vi "Main_MHM01.vi"() -> ()   [LabVIEW 2013]
uses:
  <vilib>/Platform/TimedLoop/XDataNode/timing_clust.ctl
  <vilib>/Platform/TimedLoop/XDataNode/nitl_modes.ctl
  <vilib>/Platform/TimedLoop/XDataNode/wakeup.ctl
  <vilib>/platform/TimedLoop/XDataNode/XDataNode.xnode
  <vilib>/Platform/TimedLoop/XDataNode/XDNodeRunTimeDep.lvlib
panel:
  out "Export Folder Path":path
  in  "DO select":dbl[](array[numeric])
  in  "Names legend":string[](array[string])=["s1", "s2"]
  out "Unit display A":dbl[][](graph)=[[528.1875, 527.4375, 528.1875, 527.25, 525.75, 520.125, 579.0, 800.8125, 526.6875, 524.25, 525.0, 525.1875]]
  in  "Period (ms)":i64=1000
  out "DO indicator":bool[](array[boolean])
  in  "AI select":dbl[](array[numeric])
  out "Sample number":u32
  in  "Stop Button":bool
  # "SELECT DO AND AI FOR EACH SENSOR"
  # "DATA folder in VI location must be created manually"
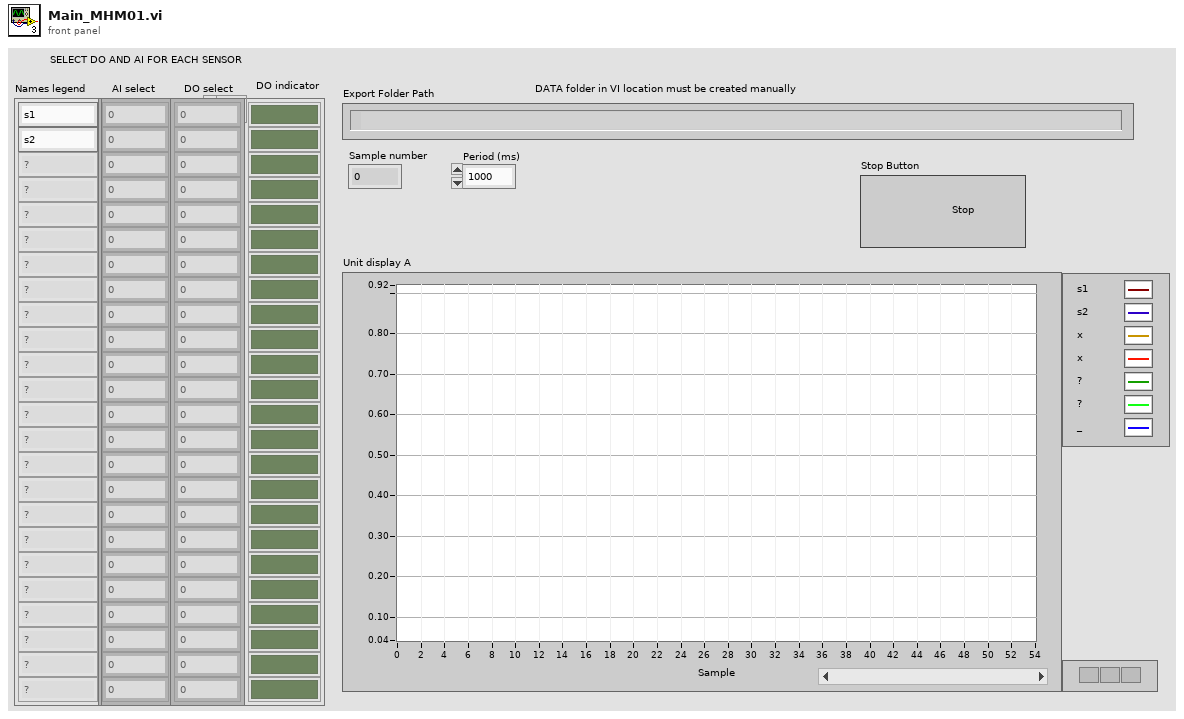
[diagram p1: front panel]
types:
  T1 = typedef "XDNodeRunTimeDep.lvlib/timing_clust.ctl" = cluster{"Expected End [f-1]":u64, "Actual End [f-1]":u64, "Finished Late? [f-1]":bool, "Expected End [i-1]":u64, "Actual End [i-1]":u64, "Finished Late? [i-1]":bool, "Expected Start [i]":u64, "Actual Start [i]":u64, "Expected Start [f]":u64, "Actual Start [f]":u64, "Source Name":string, "Structure Name":string, "Period":i64, "Deadline":i64, "Offset":i64, "Start":i64, "Priority":i32, "Timeout":i32, "Mode":T2, "Wakeup Reason":T3, "Error":errorcluster, "Source Type":string, "Secondary Source Type":string, "Global End Time":u64, "Global Start Time":u64, "Frame Duration":u64, "Iteration Duration":u64, "Assigned CPU":i32, "I/O Scan Engine Mode":u32}
  T2 = typedef "XDNodeRunTimeDep.lvlib/nitl_modes.ctl" = enum32{"No Change", "Process missed periods, maintain original phase", "Discard missed periods, maintain original phase", "Process missed periods, ignore original phase", "Discard missed periods, ignore original phase"}
  T3 = typedef "XDNodeRunTimeDep.lvlib/wakeup.ctl" = enum32{"Normal", "Aborted", "Asynchronous wakeup", "Timing source error", "Timed loop error", "Timeout"}
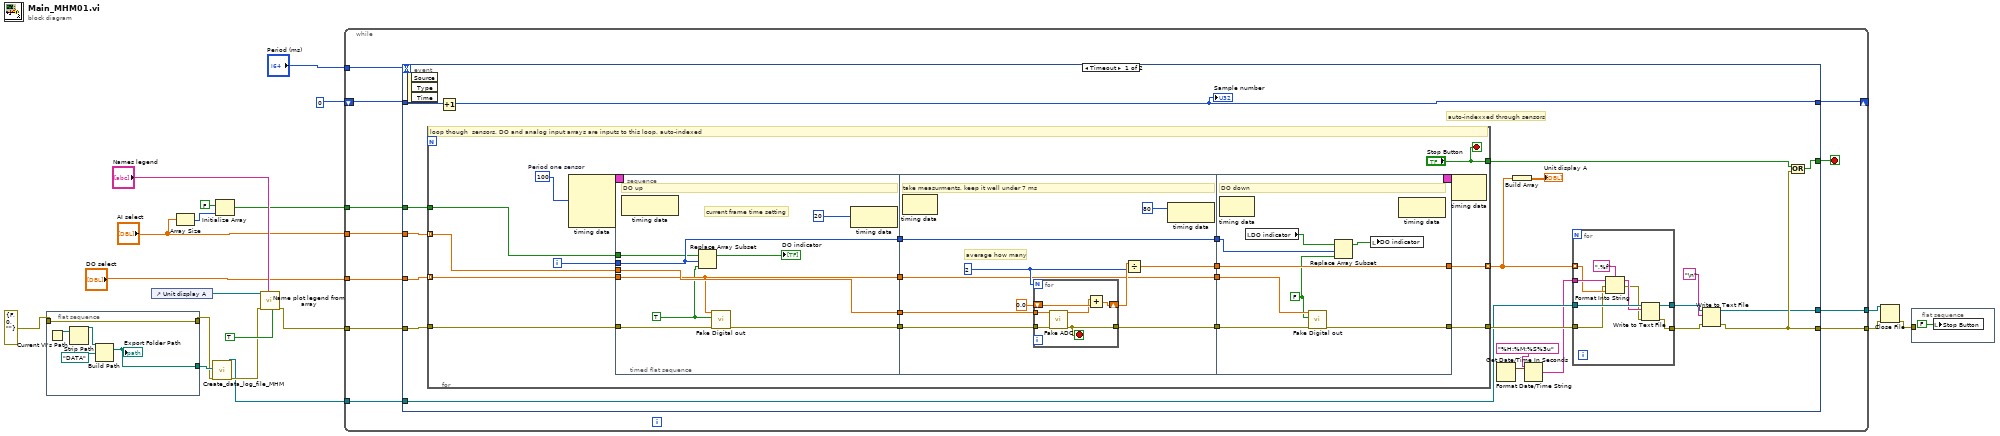
[diagram p0: block diagram]
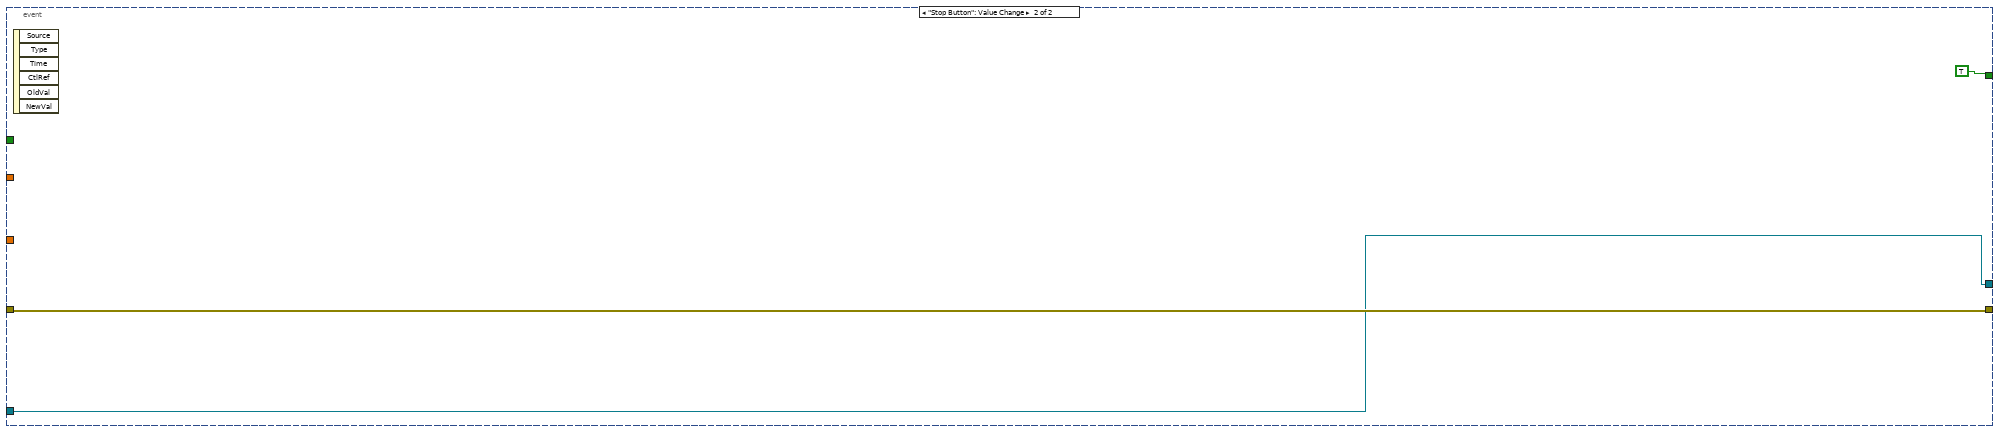
[diagram p2: hidden frame]
diagram:
  n1 = flat-sequence {
    tunnel: errorcluster {"status"=FALSE, "code"=0, "source"=""} ("error constant") -> [w21]
    tunnel: [w21] -> w6
    tunnel: [w20] -> w7
    frame #0 {
      n2 = Current VI's Path() -> (path=w22:path)
      n3 = Strip Path(path=w22) -> (stripped path=w23:path)  [unwired: 1 out]
      n4 = Build Path(base path=w23, name or relative path=path "DATA") -> (appended path=w20:path)
      "Export Folder Path" <- w20
    }
  }
  n5 = control-ref of="Unit display A"() -> (w14:refnum<vi>)
  n6 = Array Size(array="AI select") -> (size(s)=w10:i32)
  n7 = call "Create_data_log_file_MHM.vi"("error in (no error)"=w6, "Export Folder Path"=w7) -> ("error out"=w5:errorcluster, "Byte Stream File out"=w4:refnum<file>)  [unwired: 8 in]
  n8 = Initialize Array(FALSE, w10) -> (w9:bool[])
  n9 = call "Name plot legend from array.vi"("Force write (F)"=TRUE, "Names legend"="Names legend", "error in (no error)"=w5, "Chart in"=w14) -> ("error out"=w17:errorcluster)  [unwired: 7 in]
  n10 = while {
    tunnel: w17 -> [w35]
    tunnel: "AI select" -> [w34]
    tunnel: "DO select" -> [w33]
    tunnel: [w31] -> w3
    tunnel: "Period (ms)" -> [w30]
    shift-right: [w28] -> _
    shift-left: u32 0 -> [w29]
    tunnel: w9 -> [w27]
    tunnel: w4 -> [w26]
    tunnel: [w25] -> w1
    stop <- w32 stop-if-true
    n11 = event shown="[0] Timeout" {
      selector: _ -> [_ _]
      dyn-events: _ -> [_ _]
      timeout: w30 -> [_ _]
      tunnel: w35 -> [w55 w139]
      tunnel: w34 -> [w54 _]
      tunnel: w33 -> [w53 _]
      tunnel: [w41 TRUE] -> w32
      tunnel: [w39 w139] -> w31
      tunnel: w29 -> [w52 _]
      tunnel: [w51 _] -> w28
      tunnel: w27 -> [w49 _]
      tunnel: w26 -> [w47 w138]
      tunnel: [w36 w138] -> w25
      event Timeout {
        # "auto-indexxed through sensors"
        n12 = event-data() -> ()  [unwired: 1 in, 3 out]
        n13 = for {
          tunnel: w55 -> [w73]
          tunnel: [w71] -> w43 mode=indexing
          tunnel: w54 -> [w70] mode=indexing
          tunnel: w53 -> [w69] mode=indexing
          tunnel: ["Stop Button"] -> w40
          tunnel: [w67] -> w48
          tunnel: w49 -> [w65]
          i -> [w66]
          stop <- "Stop Button" stop-if-true
          w72 = i64 100  # Period one sensor
          # "loop though  sensors, DO and analog input arrays are inputs to this loop, auto-indexed"
          n14 = node-c288(w72) -> (w75:T1)  [unwired: 3 in]
          n15 = timed-sequence {
            timing: w75 -> [_]
            timing-out: [_] -> w74
            tunnel: w73 -> [w89]
            tunnel: [w86] -> w71
            tunnel: w70 -> [w85]
            tunnel: w69 -> [w83]
            tunnel: [w82] -> w67
            tunnel: w66 -> [w79]
            tunnel: w65 -> [w76]
            n16 = timed-flat-sequence {
              tunnel: [w96] -> w90
              tunnel: w89 -> [w97]
              tunnel: w85 -> [w98]
              tunnel: [w98] -> w84
              tunnel: w83 -> [w95]
              tunnel: [w95] -> w81
              tunnel: w79 -> [w93]
              tunnel: [w93] -> w78
              tunnel: w76 -> [w91]
              tunnel: w90 -> [w112]
              tunnel: [w111] -> w88
              tunnel: [w107] -> w87
              tunnel: w84 -> [w106]
              tunnel: w81 -> [w105]
              tunnel: [w105] -> w80
              tunnel: w78 -> [w104]
              tunnel: [w104] -> w77
              tunnel: w88 -> [w130]
              tunnel: w87 -> [w131]
              tunnel: [w131] -> w86
              tunnel: [w129] -> w82
              tunnel: w80 -> [w128]
              tunnel: w77 -> [w127]
              frame #0 {
                w92 = TRUE
                # "current frame time setting"
                # "DO up"
                n17 = node-c288() -> ()  [unwired: 1 in, 1 out]
                n18 = Replace Array Subset(array=w91, new element=w92, index=w93) -> (→"DO indicator":bool[])
                n19 = call "Fake Digital out.vi"("error in (no error)"=w97, "Value to DO"=w92, "DO select"=w95) -> ("error out"=w96:errorcluster)  [unwired: 8 in]
                n20 = node-c288(i64 20 ("Start")) -> ()  [unwired: 1 out]
              }
              frame #1 {
                w108 = 2
                # "average how many"
                # "take measurments, keep it well under 7 ms"
                n21 = node-c288() -> ()  [unwired: 1 in, 1 out]
                n22 = for {
                  N: w108 -> [_]
                  tunnel: w112 -> [w116]
                  tunnel: [w115] -> w111
                  shift-right: [w118] -> w109
                  shift-left: 0.0 -> [w119]
                  tunnel: w106 -> [w114]
                  stop <- w115 stop-if-true
                  n23 = call "Fake ADC.vi"("error in (no error)"=w116, "AI select"=w114) -> ("error out"=w115:errorcluster, "Ouptut"=w117:dbl)  [unwired: 8 in]
                  n24 = Add(x=w117, y=w119) -> (x+y=w118:dbl)
                }
                n25 = Divide(x=w109, y=w108) -> (x/y=w107:dbl)
                n26 = node-c288(i64 80 ("Start")) -> ()  [unwired: 1 out]
              }
              frame #2 {
                w125 = FALSE ("DO")
                # "DO down"
                n27 = node-c288() -> ()  [unwired: 1 in, 1 out]
                n28 = local read "DO indicator"() -> (w126:bool[])
                n29 = call "Fake Digital out.vi"("error in (no error)"=w130, "Value to DO"=w125, "DO select"=w128) -> ("error out"=w129:errorcluster)  [unwired: 8 in]
                n30 = Replace Array Subset(array=w126, new element=w125, index=w127) -> (w124:bool[])
                n31 = local write "DO indicator"(w124) -> ()
                n32 = node-c288() -> ()  [unwired: 1 in, 1 out]
              }
            }
          }
          n33 = node-c288(w74) -> ()  [unwired: 1 out]
        }
        n34 = Increment(x=w52) -> (x+1=w51:u32)
        "Sample number" <- w51
        n35 = Get Date/Time In Seconds() -> (seconds since 1Jan1904=w46:timestamp)
        n36 = Build Array(w43) -> (→"Unit display A":dbl[][])
        n37 = Format Date/Time String(time format string (%c)="%H:%M:%S%3u", seconds (now)=w46) -> (date/time string=w44:string)  [unwired: 1 in]
        n38 = for {
          tunnel: w48 -> [w57]
          tunnel: [w64] -> w42
          tunnel: w47 -> [w63]
          tunnel: w44 -> [w61]
          tunnel: w43 -> [w59] mode=indexing
          tunnel: [w58] -> w38
          n39 = Format Into String(format string=",%f", initial string=w61, error in=w57, w59) -> (resulting string=w62:string, error out=w56:errorcluster)
          n40 = Write to Text File(file (use dialog)=w63, text=w62, error in=w56) -> (refnum out=w58:refnum<file>, error out=w64:errorcluster)  [unwired: 1 in, 1 out]
        }
        n41 = Write to Text File(file (use dialog)=w38, text="\n", error in=w42) -> (refnum out=w36:refnum<file>, error out=w39:errorcluster)  [unwired: 1 in, 1 out]
        n42 = Or(x=w40, y=w39) -> (x .or. y?=w41:bool)
      }
      event "Stop Button": Value Change {
        n43 = event-data() -> ()  [unwired: 1 in, 6 out]
      }
    }
  }
  n44 = Close File(refnum=w1, error in=w3) -> (error out=w2:errorcluster)  [unwired: 1 out]
  n45 = flat-sequence {
    tunnel: w2 -> [_]
    frame #0 {
      n46 = local write "Stop Button"(FALSE ("Stop Button")) -> ()
    }
  }
